vi "故障告警日志存储 (子VI).vi"(6 "故障代码":u16, 7 "告警代码":u16, 9 "日志代码":u16, 10 "参数":string, 11 "队列输入":refnum<queue>) -> ()   [LabVIEW 2016, in "斯坦道CODMn新电路板.lvlib"]
uses:
  Alarm interface/Alarm interface.lvlib
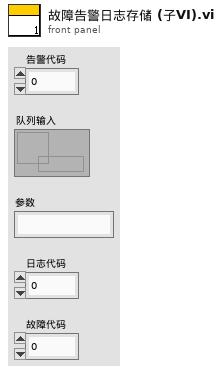
[diagram p1: front panel]
types:
  T1 = cluster{"id":string, "code":i32, "level":enum16{"一级", "二级", "三级"}, "message":string, "analysis":string, "platform_alarm_code":string}
  T2 = typedef "报警信息字段定义.ctl" = cluster{"时间":timestamp, "参数":string, "报警信息":string, "备注":string, "code":u64, "platform_alarm_code":string}
  T3 = cluster{"id":string, "ver":string, "type":string, "code":u16, "level":enum16{"一级", "二级", "三级"}, "message":string, "analysis":string, "platform_alarm_code":string}
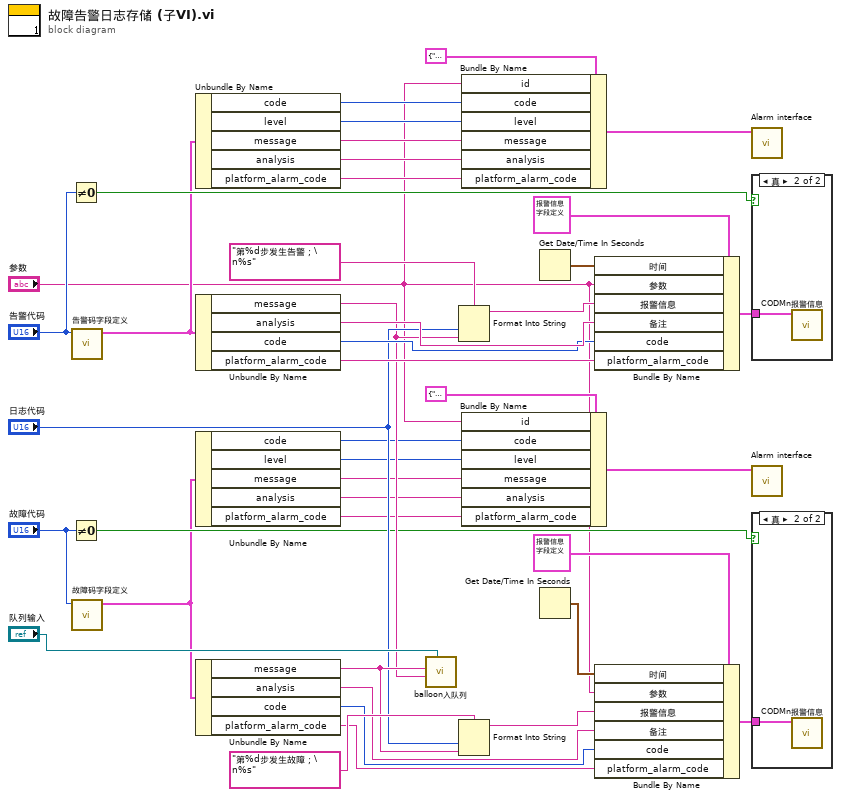
[diagram p0: block diagram]
diagram:
  n1 = Not Equal To 0?(x="告警代码") -> (x != 0?=w20:bool)
  n2 = Not Equal To 0?(x="故障代码") -> (x != 0?=w18:bool)
  n3 = call "告警码字段定义.vi"("告警代码"="告警代码") -> ("报警信息"=w11:T3)  [unwired: 10 in]
  n4 = call "故障码字段定义.vi"("故障代码"="故障代码") -> ("故障信息"=w2:T3)  [unwired: 10 in]
  n5 = Unbundle By Name(w11) -> ("code"=w17:u16, "level"=w16:enum16{"一级", "二级", "三级"}, "message"=w15:string, "analysis"=w14:string, "platform_alarm_code"=w13:string)
  n6 = Unbundle By Name(w11) -> ("message"=w22:string, "analysis"=w27:string, "code"=w26:u16, "platform_alarm_code"=w25:string)
  n7 = Unbundle By Name(w2) -> ("code"=w9:u16, "level"=w8:enum16{"一级", "二级", "三级"}, "message"=w7:string, "analysis"=w6:string, "platform_alarm_code"=w5:string)
  n8 = Unbundle By Name(w2) -> ("message"=w28:string, "analysis"=w31:string, "code"=w30:u16, "platform_alarm_code"=w29:string)
  n9 = call "balloon入队列.vi"("队列"="队列输入", "告警信息"=w22, "故障信息"=w28) -> ()  [unwired: 8 in, 1 out]
  n10 = Format Into String(format string="第%d步发生告警；\n%s" ("格式字符串"), "日志代码", w22) -> (resulting string=w23:string)  [unwired: 2 in, 1 out]
  n11 = Format Into String(format string="第%d步发生故障；\n%s" ("格式字符串"), "日志代码", w28) -> (resulting string=w32:string)  [unwired: 2 in, 1 out]
  n12 = Bundle By Name(cluster=T1 {"id"="", "code"=0, "level"=enum."一级", "message"="", "analysis"="", "platform_alarm_code"=""} ("簇"), "id"="参数", "code"=w17, "level"=w16, "message"=w15, "analysis"=w14, "platform_alarm_code"=w13) -> (w10:T1)
  n13 = Bundle By Name(cluster=T1 {"id"="", "code"=0, "level"=enum."一级", "message"="", "analysis"="", "platform_alarm_code"=""} ("簇"), "id"="参数", "code"=w9, "level"=w8, "message"=w7, "analysis"=w6, "platform_alarm_code"=w5) -> (w3:T1)
  n14 = Get Date/Time In Seconds() -> (seconds since 1Jan1904=w33:timestamp)
  n15 = Get Date/Time In Seconds() -> (seconds since 1Jan1904=w39:timestamp)
  n16 = Bundle By Name(cluster=T2 {"时间"=timestamp(0 s since 1904-01-01), "参数"="", "报警信息"="", "备注"="", "code"=0, "platform_alarm_code"=""} ("data"), "时间"=w33, "参数"="参数", "报警信息"=w23, "备注"=w27, "code"=w26, "platform_alarm_code"=w25) -> (w35:T2)
  n17 = Bundle By Name(cluster=T2 {"时间"=timestamp(0 s since 1904-01-01), "参数"="", "报警信息"="", "备注"="", "code"=0, "platform_alarm_code"=""} ("data"), "时间"=w39, "参数"="参数", "报警信息"=w32, "备注"=w31, "code"=w30, "platform_alarm_code"=w29) -> (w38:T2)
  n18 = call "Alarm interface.vi"("簇"=w10) -> ()  [unwired: 10 in, 1 out]
  n19 = case shown="真" w20 {
    tunnel: w35 -> [_ w42]
    frame False {
    }
    frame True {
      n20 = call "CODMn报警信息.vi"("data"=w42) -> ()  [unwired: 10 in, 1 out]
    }
  }
  n21 = call "Alarm interface.vi"("簇"=w3) -> ()  [unwired: 10 in, 1 out]
  n22 = case shown="真" w18 {
    tunnel: w38 -> [_ w43]
    frame False {
    }
    frame True {
      n23 = call "CODMn报警信息.vi"("data"=w43) -> ()  [unwired: 10 in, 1 out]
    }
  }
